vi "Meas Result Generate TWM Digitizer Correction - Process Measurement.vi"(4 "Estimate non-linearity (False)":bool, 5 "digitizer type":T1=enum."HP3458A", 6 "use aperture correction (true)":bool=TRUE, 7 "table ref":refnum<vi>, 8 "error in":errorcluster, 9 "use time shift (true)":bool=TRUE, 10 "Mode":T3, 11 "meas":T4={"swp cfg"={"N"=0, "R"=0, "f list"=[], "smpl delay"=0.0, "set delay"=0.0, "set delay np"=0.0, "meas root"=path "", "meas name"="", "meas a-index"=FALSE, "rnd sweep"=FALSE, "mode"=enum."Frequency", "swp mode"=enum."Linear", "avg"=0, "subrec"=0, "multi-freq"=FALSE}, "bridge"={"type"=enum."TWM client", "TWM"={"pipe name"="", "parameters"=[], "handle"=0, "fixed aper [s]"=0.0, "f-list [Hz]"=[], "discrete f-list"=FALSE, "unc mode"=enum."None", "unc mcc"=0, "unc first"=FALSE}, "last f"=0.0, "bias comp"={"bias type"=enum."dummy", "VISA"="", "Enable"=FALSE, "channel qu"=[], "channel Uinit"=[]}, "sim mode"=enum."Generic RLC network", "channel idns"=[], "sim phases"=1}, "src"={"type"=enum."Tektronix AFG3101C", "afg"={"VISA"="", "const"=0.0, "gen DC"=FALSE, "ext ref"=FALSE}, "cDAQ dds"={"device"="", "channels"=[], "mclk source"="", "mclk [Hz]"=0.0, "fs [Hz]"=0.0, "block [s]"=0.0, "buf [s]"=0.0, "task"="", "cmd queue"=refnum, "proc ref"=refnum, "smpl clock out"="/cDAQ3/PFI0", "export smpl clock"=FALSE, "DC ofs [V]"=[], "timebase source"="", "timebase mode"=enum."Local"}, "gain [V/A]"=1.0, "F5xxx session"={"VISA"="", "mode"=enum."AC voltage", "Earth on"=FALSE, "Ext ref lock"=FALSE}}, "results"=refnum} {"src"."cDAQ dds"."channels" min=0 step=1; "bridge"."TWM"."f-list [Hz]" format="%#_6p"; "swp cfg"."f list"."bias" format="%#_3p"; "swp cfg"."f list"."level" format="%#_3p"; "swp cfg"."f list"."fs [Hz]" format="%#_5p"; "swp cfg"."f list"."time [s]" format="%#_3p"; "swp cfg"."f list"."f/fs" format="%#_3p"; "swp cfg"."f list"."periods" format="%#_3f"; "swp cfg"."f list"."f [Hz]" format="%#_5p"}) -> (0 "error out":errorcluster, 3 "correction data":T2)   [LabVIEW 2020]
doc: "Generates simple TWM digitizer correction from measured data."
uses:
  meas session.ctl
  Meas Sweep Config.ctl
  Meas Freq Info.ctl
  meas_swp_mode.ctl
  meas_sweep_flist_mode.ctl
  bridge/Bridge Session.ctl
  bridge/Bridge Type.ctl
  drivers/TWM client/TWM Session.ctl
  drivers/TWM client/TWM parameters.ctl
  drivers/TWM client/Meas Proc QWTB Uncertainty Mode.ctl
  bridge/Bridge Bias Session.ctl
  bridge/Bridge Bias Type.ctl
  bridge/Bridge Sim Mode.ctl
  source/Source Session.ctl
  source/Source Type.ctl
  drivers/AFG3101C/AFG3101C Session.ctl
  drivers/cDAQ DDS/cDAQ DDS Session.ctl
  drivers/cDAQ DDS/cDAQ DDS Setup.ctl
  drivers/cDAQ DDS/cDAQ DDS Timebase Mode.ctl
  drivers/Fluke 5XXX/top_lev/F5xxx_session.ctl
  drivers/Fluke 5XXX/top_lev/F5xxx_output_mode.ctl
  Meas Results Ref.ctl
  Meas Results.ctl
  bridge/Bridge Frequency Readings Data.ctl
  drivers/TWM client/Meas Proc QWTB Spectrum Data.ctl
  drivers/TWM client/TWM Phase Info.ctl
  Meas Results Correction Structuring Mode.ctl
  Meas Results TWM Digitizer Correction Data.ctl
  Meas Results TWM Correction Digitizer Type.ctl
  Meas Results Sweep Data Uncertainty Mode.ctl
panel:
  out "time shifts [s]":dbl[][](array[numeric]) format="%#_6p"
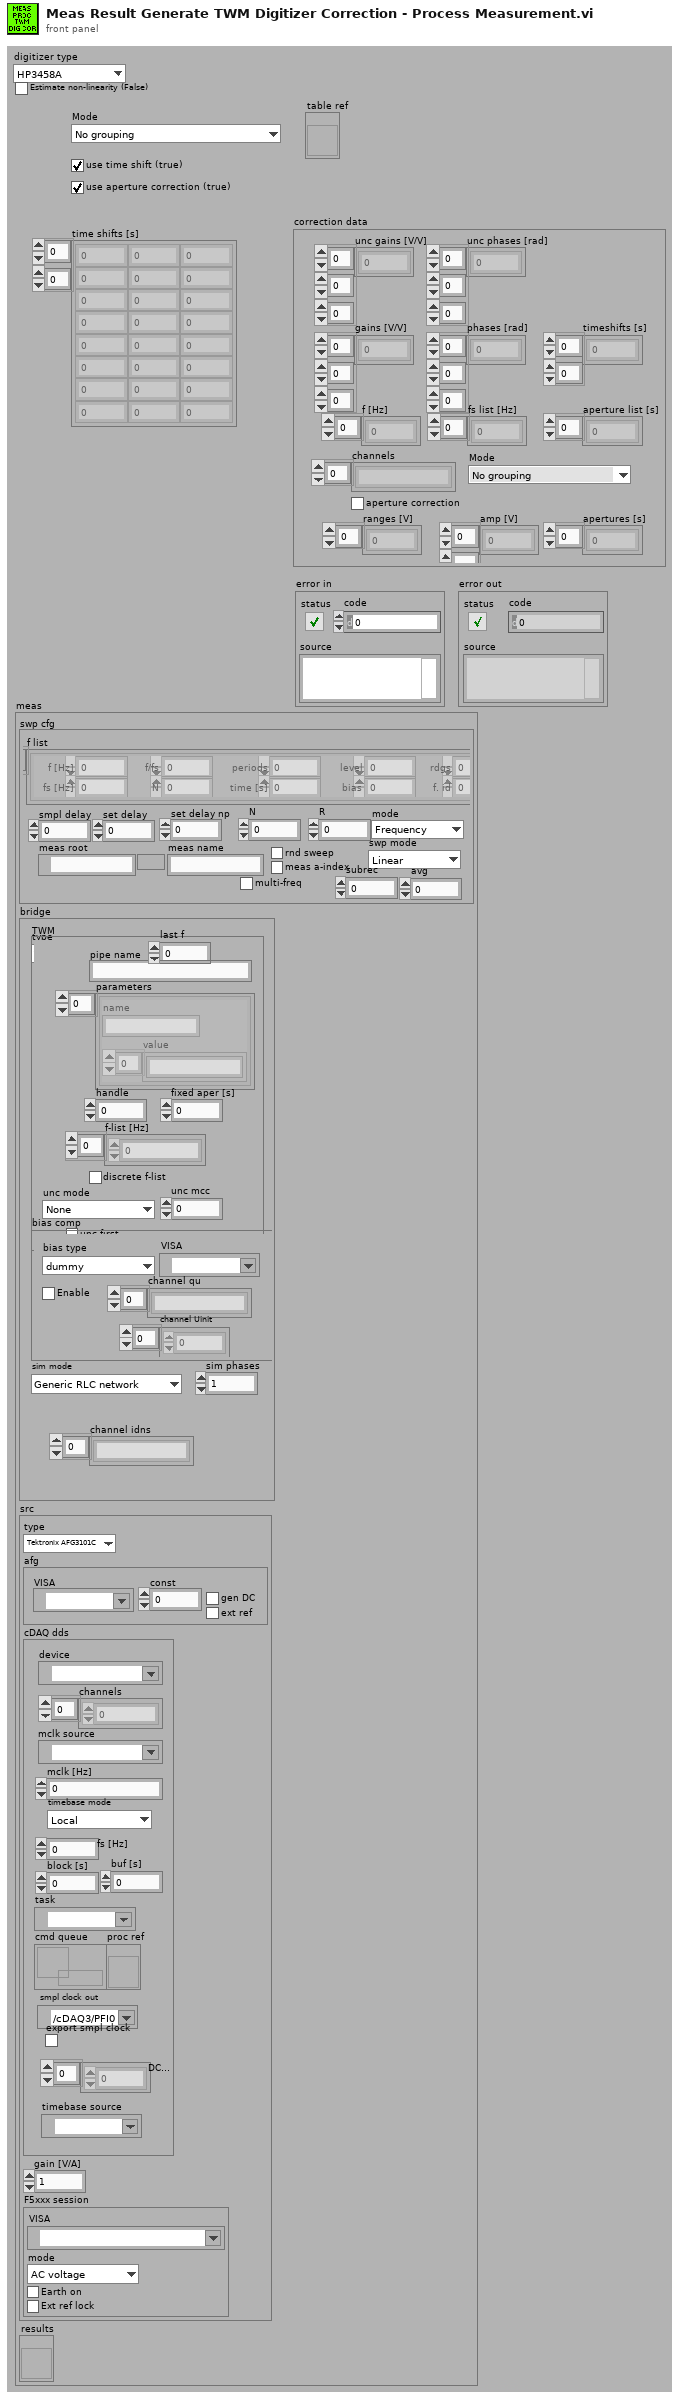
[diagram p1: front panel]
types:
  T1 = typedef "Meas Results TWM Correction Digitizer Type.ctl" = enum16{"Unknown", "HP3458A", "NI9238"}
  T2 = typedef "Meas Results TWM Digitizer Correction Data.ctl" = cluster{"gains [V/V]":dbl[][][], "phases [rad]":dbl[][][], "timeshifts [s]":dbl[][], "f [Hz]":dbl[], "fs list [Hz]":dbl[], "aperture list [s]":dbl[], "channels":string[], "Mode":T3, "aperture correction":bool, "ranges [V]":dbl[], "amp [V]":dbl[][], "apertures [s]":dbl[], "unc gains [V/V]":dbl[][][], "unc phases [rad]":dbl[][][]}
  T3 = typedef "Meas Results Correction Structuring Mode.ctl" = enum16{"No grouping", "Group by apertures (3458A)", "Group by fs (generic digitizer)"}
  T4 = typedef "meas session.ctl" = cluster{"swp cfg":T5, "bridge":T9, "src":T17, "results":T24}
  T5 = typedef "Meas Sweep Config.ctl" = cluster{"N":i32, "R":i32, "f list":T6[], "smpl delay":dbl, "set delay":dbl, "set delay np":dbl, "meas root":path, "meas name":string, "meas a-index":bool, "rnd sweep":bool, "mode":T7, "swp mode":T8, "avg":i32, "subrec":i32, "multi-freq":bool}
  T6 = typedef "Meas Freq Info.ctl" = cluster{"f [Hz]":dbl, "periods":dbl, "f/fs":dbl, "time [s]":dbl, "fs [Hz]":dbl, "N":i32, "level":dbl, "bias":dbl, "rdgs":i32, "f. id":i32}
  T7 = typedef "meas_swp_mode.ctl" = enum16{"Frequency", "Level", "Bias"}
  T8 = typedef "meas_sweep_flist_mode.ctl" = enum16{"Linear", "Log10"}
  T9 = typedef "Bridge Session.ctl" = cluster{"type":T10, "TWM":T11, "last f":dbl, "bias comp":T14, "sim mode":T16, "channel idns":string[], "sim phases":i32}
  T10 = typedef "Bridge Type.ctl" = enum16{"TWM client", "dummy"}
  T11 = typedef "TWM Session.ctl" = cluster{"pipe name":string, "parameters":T12[], "handle":i32, "fixed aper [s]":dbl, "f-list [Hz]":dbl[], "discrete f-list":bool, "unc mode":T13, "unc mcc":i32, "unc first":bool}
  T12 = typedef "TWM parameters.ctl" = cluster{"name":string, "value":string[]}
  T13 = typedef "Meas Proc QWTB Uncertainty Mode.ctl" = enum16{"None", "GUF", "Monte Carlo"}
  T14 = typedef "Bridge Bias Session.ctl" = cluster{"bias type":T15, "VISA":refnum<visa-resource-name>, "Enable":bool, "channel qu":string[], "channel Uinit":dbl[]}
  T15 = typedef "Bridge Bias Type.ctl" = enum16{"dummy", "CMI LiBbias V1.0"}
  T16 = typedef "Bridge Sim Mode.ctl" = enum16{"Generic RLC network", "Interchannel transfer"}
  T17 = typedef "Source Session.ctl" = cluster{"type":T18, "afg":T19, "cDAQ dds":T20, "gain [V/A]":dbl, "F5xxx session":T22}
  T18 = typedef "Source Type.ctl" = enum16{"Tektronix AFG3101C", "cDAQ DAC", "Fluke 5xxx", "Agilent 33120A", "dummy"}
  T19 = typedef "AFG3101C Session.ctl" = cluster{"VISA":refnum<visa-resource-name>, "const":dbl, "gen DC":bool, "ext ref":bool}
  T20 = typedef "cDAQ DDS Session.ctl" = cluster{"device":tag, "channels":i32[], "mclk source":tag, "mclk [Hz]":dbl, "fs [Hz]":dbl, "block [s]":dbl, "buf [s]":dbl, "task":refnum<k21>, "cmd queue":refnum<queue>, "proc ref":refnum<vi>, "smpl clock out":tag, "export smpl clock":bool, "DC ofs [V]":dbl[], "timebase source":tag, "timebase mode":T21}
  T21 = typedef "cDAQ DDS Timebase Mode.ctl" = enum16{"Local", "Take from ADC (e.g. NI 9238)", "Other source"}
  T22 = typedef "F5xxx_session.ctl" = cluster{"VISA":refnum<visa-resource-name>, "mode":T23, "Earth on":bool, "Ext ref lock":bool}
  T23 = typedef "F5xxx_output_mode.ctl" = enum16{"AC voltage", "AC current"}
  T24 = typedef "Meas Results Ref.ctl" = refnum<vi>
  T25 = typedef "Meas Results Sweep Data Uncertainty Mode.ctl" = enum16{"ua(y)", "ua(y) (p=95%)", "uc(y) (p=95%)"}
  T26 = typedef "Meas Results.ctl" = cluster{"freqs":T27[][], "locked":bool, "last fid":i32, "modified":bool, "mjr name":string, "mnr name":string, "last spectra":T28[][], "saved?":bool, "TWM phase":T29[], "time start":timestamp, "time stop":timestamp}
  T27 = typedef "Bridge Frequency Readings Data.ctl" = cluster{"Udut":dbl[], "Iref":dbl[], "Udc":dbl[], "Idc":dbl[], "mjr":dbl[], "mnr":dbl[], "mjr_sh":dbl[], "mnr_sh":dbl[], "u(mjr)":dbl[], "u(mnr)":dbl[], "ua2(mjr)":dbl[], "ua2(mnr)":dbl[], "n":i32, "f [Hz]":dbl, "fs [Hz]":dbl, "aperture [s]":dbl}
  T28 = typedef "Meas Proc QWTB Spectrum Data.ctl" = cluster{"x":sgl[], "y":sgl[], "label":string}
  T29 = typedef "TWM Phase Info.ctl" = cluster{"ref chn id (I)":string, "dut chn id (U)":string, "ref chn range [V]":dbl, "dut chn range [V]":dbl, "aperture [s]":dbl, "fs [Hz]":dbl, "ref chn transducer (I)":string, "dut chn transducer (U)":string}
  T30 = typedef "Meas Results Sweep Data.ctl" = cluster{"Udut":dbl[], "Iref":dbl[], "Udc":dbl[], "Idc":dbl[], "mjr":dbl[], "mnr":dbl[], "mjr_sh":dbl[], "mnr_sh":dbl[], "f [Hz]":dbl[], "n [-]":i32[], "fs [Hz]":dbl[], "aperture [s]":dbl[]}
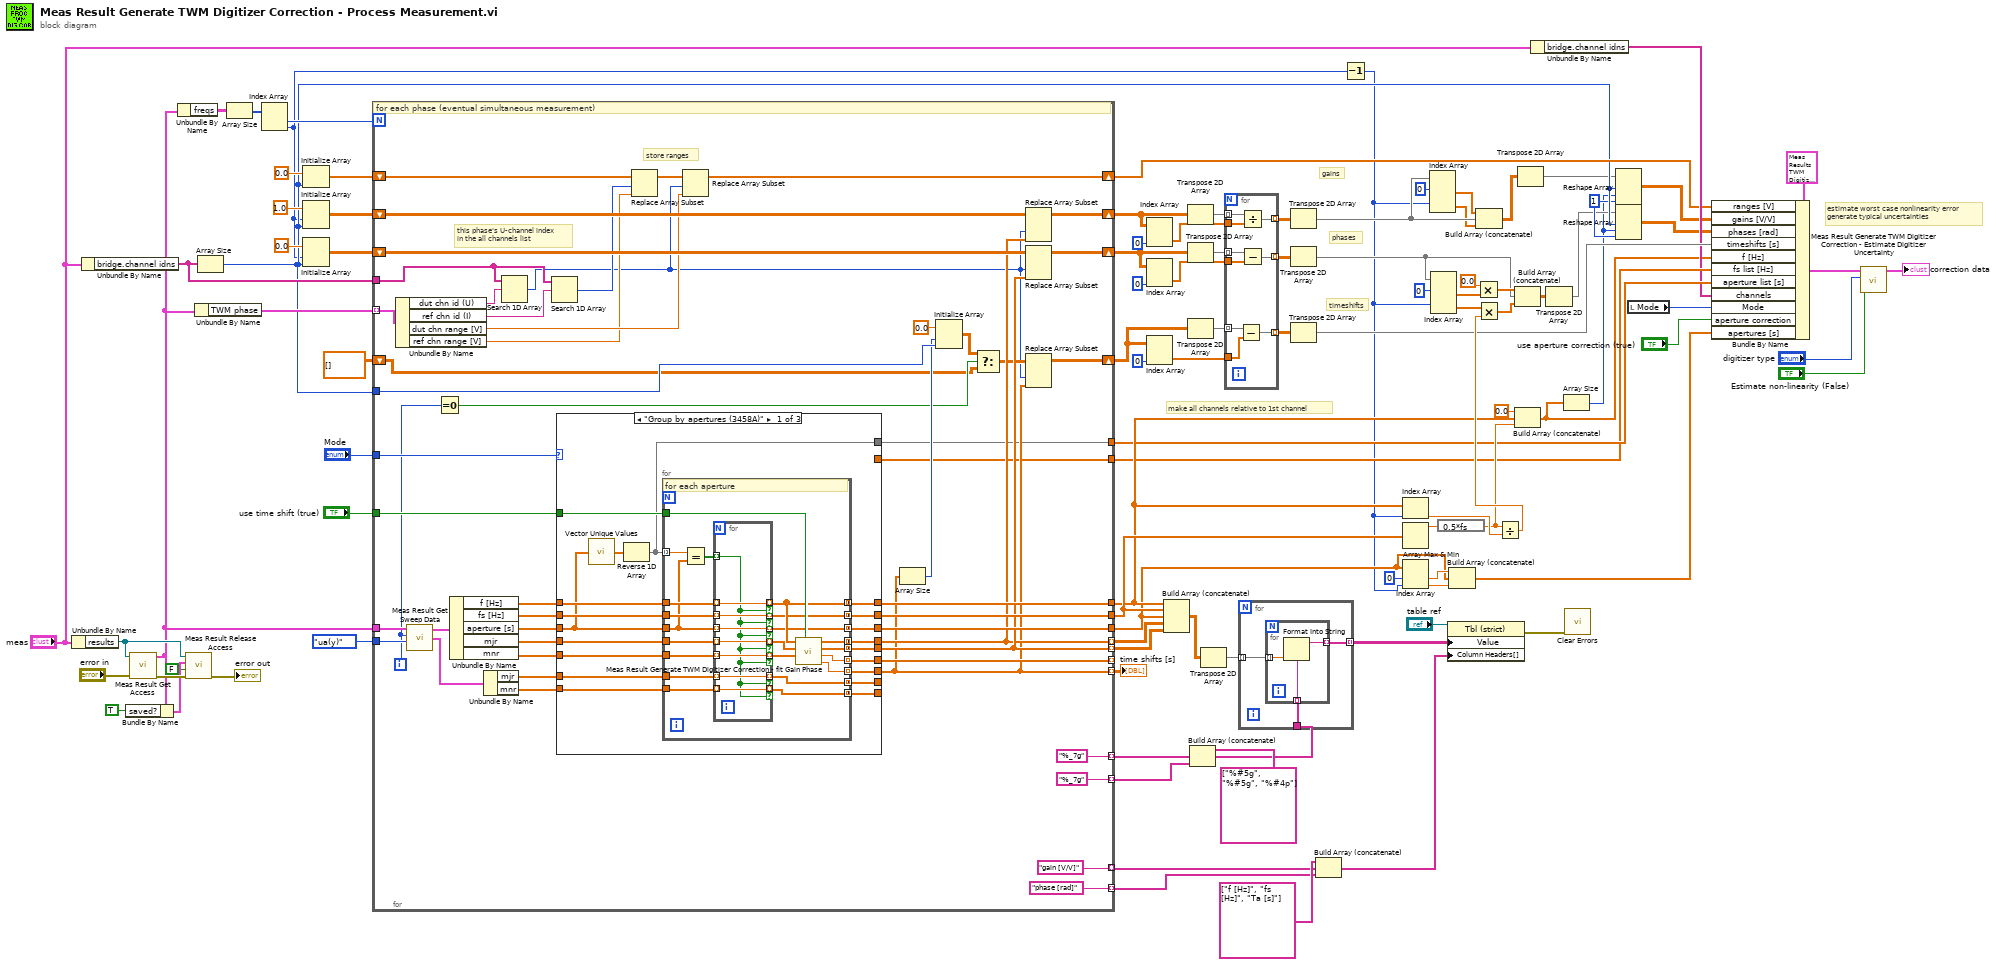
[diagram p0: block diagram]
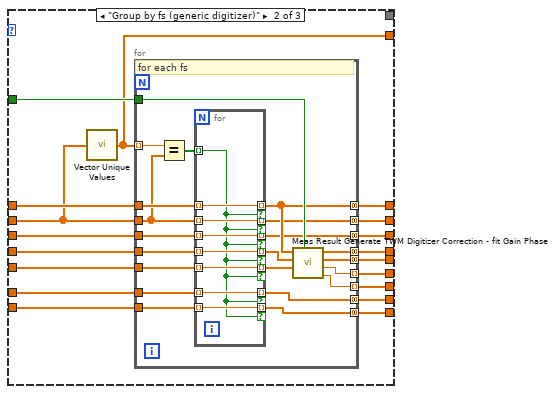
[diagram p2: hidden frame]
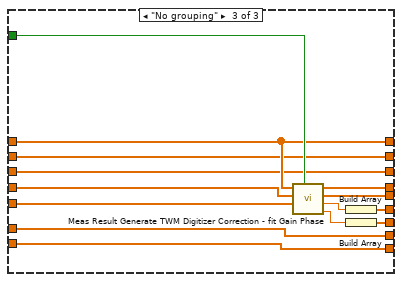
[diagram p3: hidden frame]
diagram:
  w9 = 1 ("dimension size")
  # "estimate worst case nonlinearity error\ngenerate typical uncertainties"
  # "timeshifts"
  # "phases"
  # "gains"
  # "make all channels relative to 1st channel"
  n1 = Unbundle By Name("meas") -> ("results"=w95:T24)
  n2 = Unbundle By Name("meas") -> ("bridge.channel idns"=w78:string[])
  n3 = call "Meas Result Get Access.vi"("error in"="error in", "results ref"=w95) -> ("error out"=w98:errorcluster, "results data"=w77:T26)  [unwired: 8 in]
  n4 = Bundle By Name(cluster=w77, "saved?"=TRUE) -> (w96:T26)
  n5 = Unbundle By Name(w77) -> ("freqs"=w101:T27[][])
  n6 = call "Meas Result Release Access.vi"("error in"=w98, "Release only (True)"=FALSE, "results data in"=w96, "results ref"=w95) -> ("error out"=→"error out":errorcluster)  [unwired: 7 in]
  n7 = Unbundle By Name(w77) -> ("TWM phase"=w76:T29[])
  n8 = Array Size(array=w78) -> (size(s)=w12:i32)
  n9 = Array Size(array=w101) -> (size(s)=w100:i32[])
  n10 = Index Array(array=w100) -> (element #1=w99:i32, element #2=w10:i32)  [unwired: 2 in]
  n11 = Initialize Array(0.0 ("element"), w12) -> (w23:dbl[])
  n12 = Initialize Array(1.0 ("element"), w10, w12) -> (w74:dbl[][])
  n13 = Initialize Array(0.0 ("element"), w10, w12) -> (w79:dbl[][])
  n14 = for {
    N: w99 -> [_]
    tunnel: Meas_Results_Sweep_Data_Uncertainty_Mode."ua(y)" ("uncertainty mode") -> [w151]
    tunnel: w77 -> [w136]
    tunnel: "Mode" -> [w150]
    tunnel: "use time shift (true)" -> [w145]
    tunnel: [w144] -> w40
    tunnel: [w143] -> w49
    tunnel: [w142] -> w18
    tunnel: [w131] -> w87 mode=indexing
    tunnel: [w137] -> w86 mode=indexing
    tunnel: [w128] -> _ mode=indexing
    tunnel: [w120] -> w81 mode=indexing
    tunnel: ["%_7g"] -> w84 mode=indexing
    tunnel: ["%_7g"] -> w83 mode=indexing
    shift-right: [w138] -> w69
    shift-left: w79 -> [w139]
    tunnel: w78 -> [w110]
    tunnel: w76 -> [w135] mode=indexing
    shift-right: [w133] -> w72
    shift-left: w74 -> [w132]
    shift-right: [w121] -> w63
    shift-left: dbl[][] [] -> [w123]
    tunnel: w12 -> [w129]
    tunnel: [w119] -> w37
    tunnel: [w118] -> w36
    tunnel: ["gain [V/V]"] -> w30 mode=indexing
    tunnel: ["phase [rad]"] -> w29 mode=indexing
    shift-right: [w111] -> w22
    shift-left: w23 -> [w107]
    i -> [w126]
    # "store ranges"
    # "this phase's U-channel index\nin the all channels list"
    # "for each phase (eventual simultaneous measurement)"
    n15 = Unbundle By Name(w135) -> ("dut chn id (U)"=w134:string, "ref chn id (I)"=w109:string, "dut chn range [V]"=w105:dbl, "ref chn range [V]"=w104:dbl)
    n16 = call "Meas Result Get Sweep Data.vi"("uncertainty mode"=w151, "phase index (default: 0)"=w126, "result"=w136) -> ("unc(data)"=w114:T30, "data"=w152:T30)  [unwired: 1 in, 1 out]
    n17 = Equal To 0?(x=w126) -> (x = 0?=w125:bool)
    n18 = Unbundle By Name(w152) -> ("f [Hz]"=w149:dbl[], "fs [Hz]"=w148:dbl[], "aperture [s]"=w147:dbl[], "mjr"=w115:dbl[], "mnr"=w146:dbl[])
    n19 = Unbundle By Name(w114) -> ("mjr"=w113:dbl[], "mnr"=w112:dbl[])
    n20 = Search 1D Array(1D array=w110, element=w134) -> (index of element=w103:i32)  [unwired: 1 in]
    n21 = Search 1D Array(1D array=w110, element=w109) -> (index of element=w106:i32)  [unwired: 1 in]
    n22 = case shown="\"Group by apertures (3458A)\"" w150 {
      tunnel: w149 -> [w171 w218 w258]
      tunnel: w148 -> [w170 w213 w251]
      tunnel: w147 -> [w167 w215 w250]
      tunnel: w115 -> [w169 w217 w261]
      tunnel: w146 -> [w168 w216 w260]
      tunnel: w145 -> [w165 w214 w259]
      tunnel: [w164 w212 w258] -> w144
      tunnel: [w163 w211 w251] -> w143
      tunnel: [w162 w210 w250] -> w142
      tunnel: [w161 w209 w257] -> w131
      tunnel: [w160 w208 w256] -> w137
      tunnel: [w159 w207 w252] -> w128
      tunnel: [w158 w206 w253] -> w120
      tunnel: [w157 _ _] -> w119
      tunnel: [_ w205 _] -> w118
      tunnel: w113 -> [w156 w204 w248]
      tunnel: w112 -> [w155 w203 w249]
      tunnel: [w154 w202 w248] -> _
      tunnel: [w153 w201 w249] -> _
      frame "Group by apertures (3458A)" {
        n23 = call "Vector Unique Values.vi"("array in"=w167) -> ("uniques out"=w166:dbl[])
        n24 = Reverse 1D Array(array=w166) -> (reversed array=w157:dbl[])
        n25 = for {
          tunnel: w171 -> [w190]
          tunnel: w170 -> [w189]
          tunnel: w167 -> [w188]
          tunnel: w169 -> [w187]
          tunnel: w168 -> [w186]
          tunnel: w157 -> [w192] mode=indexing
          tunnel: w165 -> [w183]
          tunnel: [w182] -> w164 mode=concatenating
          tunnel: [w181] -> w163 mode=concatenating
          tunnel: [w180] -> w162 mode=concatenating
          tunnel: [w179] -> w161 mode=concatenating
          tunnel: [w178] -> w160 mode=concatenating
          tunnel: [w177] -> w159 mode=indexing
          tunnel: [w176] -> w158 mode=indexing
          tunnel: w156 -> [w175]
          tunnel: w155 -> [w174]
          tunnel: [w173] -> w154 mode=concatenating
          tunnel: [w172] -> w153 mode=concatenating
          # "for each aperture"
          n26 = Equal?(x=w192, y=w188) -> (x = y?=w191:bool[])
          n27 = for {
            tunnel: w191 -> [w193] mode=indexing
            tunnel: [w200] -> w182 mode=indexing if=w193
            tunnel: w190 -> [w200] mode=indexing
            tunnel: [w199] -> w181 mode=indexing if=w193
            tunnel: w189 -> [w199] mode=indexing
            tunnel: [w198] -> w180 mode=indexing if=w193
            tunnel: w188 -> [w198] mode=indexing
            tunnel: [w197] -> w185 mode=indexing if=w193
            tunnel: w187 -> [w197] mode=indexing
            tunnel: [w196] -> w184 mode=indexing if=w193
            tunnel: w186 -> [w196] mode=indexing
            tunnel: [w195] -> w173 mode=indexing if=w193
            tunnel: w175 -> [w195] mode=indexing
            tunnel: [w194] -> w172 mode=indexing if=w193
            tunnel: w174 -> [w194] mode=indexing
          }
          n28 = call "Meas Result Generate TWM Digitizer Correction - fit Gain Phase.vi"("use time shift (true)"=w183, "phase [rad]"=w184, "gain [V/V]"=w185, "f [Hz]"=w182) -> ("time shift [s]"=w176:dbl, "DC gain"=w177:dbl, "phase out [rad]"=w178:dbl[], "gain out [V/V]"=w179:dbl[])  [unwired: 4 in]
        }
      }
      frame "Group by fs (generic digitizer)" {
        n29 = call "Vector Unique Values.vi"("array in"=w213) -> ("uniques out"=w205:dbl[])
        n30 = for {
          tunnel: w218 -> [w237]
          tunnel: w213 -> [w223]
          tunnel: w215 -> [w236]
          tunnel: w217 -> [w235]
          tunnel: w216 -> [w234]
          tunnel: w205 -> [w239] mode=indexing
          tunnel: w214 -> [w231]
          tunnel: [w230] -> w212 mode=concatenating
          tunnel: [w229] -> w211 mode=concatenating
          tunnel: [w228] -> w210 mode=concatenating
          tunnel: [w227] -> w209 mode=concatenating
          tunnel: [w226] -> w208 mode=concatenating
          tunnel: [w225] -> w207 mode=indexing
          tunnel: [w224] -> w206 mode=indexing
          tunnel: w204 -> [w222]
          tunnel: w203 -> [w221]
          tunnel: [w220] -> w202 mode=concatenating
          tunnel: [w219] -> w201 mode=concatenating
          # "for each fs"
          n31 = Equal?(x=w239, y=w223) -> (x = y?=w238:bool[])
          n32 = for {
            tunnel: w238 -> [w240] mode=indexing
            tunnel: [w247] -> w230 mode=indexing if=w240
            tunnel: w237 -> [w247] mode=indexing
            tunnel: [w246] -> w229 mode=indexing if=w240
            tunnel: w223 -> [w246] mode=indexing
            tunnel: [w245] -> w228 mode=indexing if=w240
            tunnel: w236 -> [w245] mode=indexing
            tunnel: [w244] -> w233 mode=indexing if=w240
            tunnel: w235 -> [w244] mode=indexing
            tunnel: [w243] -> w232 mode=indexing if=w240
            tunnel: w234 -> [w243] mode=indexing
            tunnel: [w242] -> w220 mode=indexing if=w240
            tunnel: w222 -> [w242] mode=indexing
            tunnel: w221 -> [w241] mode=indexing
            tunnel: [w241] -> w219 mode=indexing if=w240
          }
          n33 = call "Meas Result Generate TWM Digitizer Correction - fit Gain Phase.vi"("use time shift (true)"=w231, "phase [rad]"=w232, "gain [V/V]"=w233, "f [Hz]"=w230) -> ("time shift [s]"=w224:dbl, "DC gain"=w225:dbl, "phase out [rad]"=w226:dbl[], "gain out [V/V]"=w227:dbl[])  [unwired: 4 in]
        }
      }
      frame "No grouping" {
        n34 = call "Meas Result Generate TWM Digitizer Correction - fit Gain Phase.vi"("use time shift (true)"=w259, "phase [rad]"=w260, "gain [V/V]"=w261, "f [Hz]"=w258) -> ("time shift [s]"=w254:dbl, "DC gain"=w255:dbl, "phase out [rad]"=w256:dbl[], "gain out [V/V]"=w257:dbl[])  [unwired: 4 in]
        n35 = Build Array(w255) -> (w252:dbl[])
        n36 = Build Array(w254) -> (w253:dbl[])
      }
    }
    n37 = Replace Array Subset(array=w107, new element=w104, index=w106) -> (w108:dbl[])
    n38 = Replace Array Subset(array=w108, new element=w105, index=w103) -> (w111:dbl[])
    n39 = Array Size(array=w120) -> (size(s)=w127:i32)
    n40 = Initialize Array(0.0 ("element"), w127, w129) -> (w124:dbl[][])
    n41 = Select(t=w124, s=w125, f=w123) -> (s? t:f=w122:dbl[][])
    n42 = Replace Array Subset(array=w132, new element=w131, index (col)=w103) -> (w133:dbl[][])  [unwired: 1 in]
    n43 = Replace Array Subset(array=w139, new element=w137, index (col)=w103) -> (w138:dbl[][])  [unwired: 1 in]
    n44 = Replace Array Subset(array=w122, new element=w120, index (col)=w103) -> (w121:dbl[][])  [unwired: 1 in]
  }
  "time shifts [s]" <- w81
  n45 = Index Array(array=w72, index (col)=0 ("disabled index (col)")) -> (element=w71:dbl[])  [unwired: 1 in]
  n46 = Index Array(array=w69, index (col)=0 ("disabled index (col)")) -> (element=w68:dbl[])  [unwired: 1 in]
  n47 = Index Array(array=w63, index (col)=0 ("disabled index (col)")) -> (element=w64:dbl[])  [unwired: 1 in]
  n48 = Build Array (concatenate)(w40, w49, w18, w87, w86) -> (w90:dbl[][])
  n49 = Transpose 2D Array(2D array=w72) -> (transposed array=w62:dbl[][])
  n50 = Transpose 2D Array(2D array=w69) -> (transposed array=w61:dbl[][])
  n51 = Transpose 2D Array(2D array=w63) -> (transposed array=w60:dbl[][])
  n52 = Build Array (concatenate)(string[] ["%#5g", "%#5g", "%#4p"], w84, w83) -> (w82:string[])
  n53 = Transpose 2D Array(2D array=w90) -> (transposed array=w91:dbl[][])
  n54 = for {
    tunnel: w62 -> [w270] mode=indexing
    tunnel: w71 -> [w269]
    tunnel: w61 -> [w268] mode=indexing
    tunnel: w68 -> [w267]
    tunnel: [w266] -> w58 mode=indexing
    tunnel: [w265] -> w67 mode=indexing
    tunnel: w60 -> [w264] mode=indexing
    tunnel: w64 -> [w263]
    tunnel: [w262] -> w59 mode=indexing
    n55 = Subtract(x=w264, y=w263) -> (x-y=w262:dbl[])
    n56 = Divide(x=w270, y=w269) -> (x/y=w266:dbl[])
    n57 = Subtract(x=w268, y=w267) -> (x-y=w265:dbl[])
  }
  n58 = for {
    tunnel: w91 -> [w272] mode=indexing
    tunnel: w82 -> [w273]
    tunnel: [w271] -> w27 mode=indexing
    n59 = for {
      tunnel: w273 -> [w275] mode=indexing
      tunnel: w272 -> [w276] mode=indexing
      tunnel: [w274] -> w271 mode=indexing
      n60 = Format Into String(format string=w275, w276) -> (resulting string=w274:string)  [unwired: 2 in, 1 out]
    }
  }
  n61 = Transpose 2D Array(2D array=w58) -> (transposed array=w54:dbl[][])
  n62 = Transpose 2D Array(2D array=w67) -> (transposed array=w43:dbl[][])
  n63 = Transpose 2D Array(2D array=w59) -> (transposed array=w38:dbl[][])
  n64 = Build Array (concatenate)(string[] ["f [Hz]", "fs [Hz]", "Ta [s]"], w30, w29) -> (w26:string[])
  n65 = Decrement(x=w10) -> (x-1=w11:i32)
  n66 = Index Array(array=w40, index=w11) -> (element=w47:dbl)
  n67 = Array Max & Min(array=w49) -> (max value=w48:dbl)  [unwired: 3 out]
  n68 = Index Array(array=w18, index #1=0 ("index"), index #2=w11) -> (element #1=w20:dbl, element #2=w19:dbl)
  n69 = Index Array(array=w54, index (row) #1=0 ("index (row)"), index (row) #2=w11) -> (element #1=w55:dbl[], element #2=w53:dbl[])  [unwired: 2 in]
  n70 = Index Array(array=w43, index (row) #1=0 ("index (row)"), index (row) #2=w11) -> (element #1=w51:dbl[], element #2=w46:dbl[])  [unwired: 2 in]
  n71 = expression code="0.5*fs"(w48) -> (w39:dbl)
  n72 = property class="Tbl (strict)"(reference="table ref", "Value"=w27, "Column Headers[]"=w26) -> (error out=w25:errorcluster)  [unwired: 1 in, 1 out]
  n73 = Build Array (concatenate)(w20, w18, w19) -> (w17:dbl[])
  n74 = Multiply(x=0.0 ("element"), y=w51) -> (x*y=w44:dbl[])
  n75 = Build Array (concatenate)(w55, w54, w53) -> (w16:dbl[][])
  n76 = Divide(x=w39, y=w47) -> (x/y=w45:dbl)
  n77 = Multiply(x=w46, y=w45) -> (x*y=w42:dbl[])
  n78 = Build Array (concatenate)(w44, w43, w42) -> (w13:dbl[][])
  n79 = Build Array (concatenate)(0.0 ("element"), w40, w39) -> (w2:dbl[])
  n80 = Transpose 2D Array(2D array=w16) -> (transposed array=w7:dbl[][])
  n81 = Unbundle By Name("meas") -> ("bridge.channel idns"=w34:string[])
  n82 = Transpose 2D Array(2D array=w13) -> (transposed array=w8:dbl[][])
  n83 = Array Size(array=w2) -> (size(s)=w1:i32)
  n84 = call <vilib>:"Clear Errors.vi"("error in (no error)"=w25) -> ()  [unwired: 5 in, 2 out]
  n85 = Reshape Array(w7, w12, w1, w9) -> (w15:dbl[][][])
  n86 = Reshape Array(w8, w12, w1, w9) -> (w14:dbl[][][])
  n87 = local read "Mode"() -> (w33:T3)
  n88 = Bundle By Name(cluster=T2 {"gains [V/V]"=[], "phases [rad]"=[], "timeshifts [s]"=[], "f [Hz]"=[], "fs list [Hz]"=[], "aperture list [s]"=[], "channels"=[], "Mode"=enum."No grouping", "aperture correction"=FALSE, "ranges [V]"=[], "amp [V]"=[], "apertures [s]"=[], "unc gains [V/V]"=[], "unc phases [rad]"=[]} ("correction data"), "ranges [V]"=w22, "gains [V/V]"=w15, "phases [rad]"=w14, "timeshifts [s]"=w38, "f [Hz]"=w2, "fs list [Hz]"=w36, "aperture list [s]"=w37, "channels"=w34, "Mode"=w33, "aperture correction"="use aperture correction (true)", "apertures [s]"=w17) -> (w6:T2)
  n89 = call "Meas Result Generate TWM Digitizer Correction - Estimate Digitizer Uncertainty.vi"("Estimate non-linearity (False)"="Estimate non-linearity (False)", "digitizer type"="digitizer type", "correction data in"=w6) -> ("correction data out"=→"correction data":T2)  [unwired: 8 in]
